vi "writeToXML.vi"(8 "error in (no error)":errorcluster, 10 "ClassLabel":string, 11 "MccAzElMove in":refnum<class "MccAzElMove.lvclass">) -> (0 "error out":errorcluster, 2 "XMLout":string, 3 "MccAzElMove out":refnum<class "MccAzElMove.lvclass">)   [LabVIEW 2022 SP3, in "TCSDataDefinitions.lvlib" / "TCSMountControlCommand.lvlib" / "CommandsForAzElAxes.lvlib" / "MccAzElMove.lvclass"]
uses:
  MccAzElMove.lvclass
  <userlib>/Common/UnitsAndXML/FlattenItemWithUnitToXML/FlattenPlaneAngleToXML/PlaneAngleUnit.ctl
  MccAzElMove.lvclass/MccAzElMove.ctl
  CommandsForAzElAxes.lvclass
  <userlib>/Common/UnitsAndXML/UnitsAndXML.lvlib
  <userlib>/Common/XML/XMLGenerator/XMLGenerator.lvclass
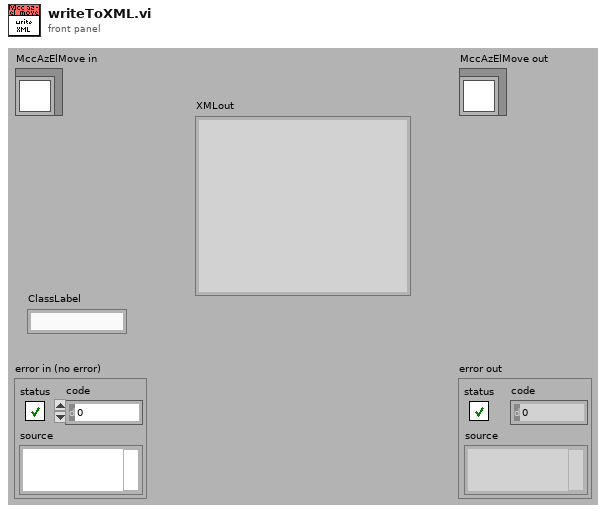
[diagram p1: front panel]
types:
  T1 = typedef "UnitsAndXML.lvlib/PlaneAngleUnit.ctl" = enum16{"rad", "deg", "'", "\""}
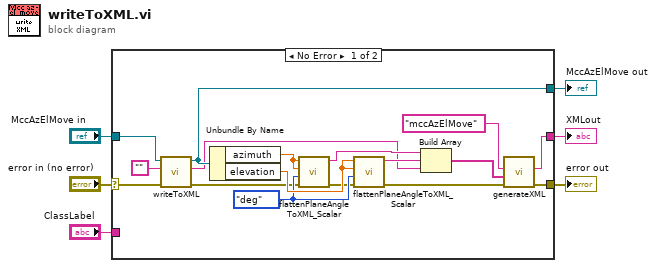
[diagram p0: block diagram]
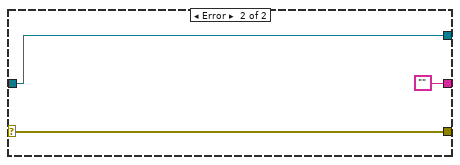
[diagram p2: hidden frame]
diagram:
  n1 = case shown="No Error" "error in (no error)" {
    selector: "error in (no error)" -> [w21 w26]
    tunnel: [w7 w26] -> w5
    tunnel: [w22 w25] -> w3
    tunnel: "MccAzElMove in" -> [w23 w25]
    tunnel: [w9 ""] -> w2
    tunnel: "ClassLabel" -> [_ _]
    frame No Error {
      w18 = PlaneAngleUnit."deg" ("planeAngleUnitInXML")
      n2 = call-parent "writeToXML.vi"("error in (no error)"=w21, "ClassLabel"="", "TCSMCCCommand in"=w23) -> ("error out"=w16:errorcluster, "XMLout"=w13:string, "TCSMCCCommand out"=w22:refnum<class "MccAzElMove.lvclass">)  [unwired: 6 in]
      n3 = Unbundle By Name(w22) -> ("azimuth"=w20:dbl[unit], "elevation"=w19:dbl[unit])
      n4 = call <userlib>:"flattenPlaneAngleToXML_Scalar.vi"("error in (no error)"=w16, "planeAngleUnitInXML"=w18, "planeAngleAgain"=w20, "planeAngle"=w20) -> ("error out"=w17:errorcluster, "xmlString"=w15:string)  [unwired: 6 in]
      n5 = call <userlib>:"flattenPlaneAngleToXML_Scalar.vi"("error in (no error)"=w17, "planeAngleUnitInXML"=w18, "planeAngleAgain"=w19, "planeAngle"=w19) -> ("error out"=w11:errorcluster, "xmlString"=w14:string)  [unwired: 6 in]
      n6 = Build Array(w15, w14, w13) -> (w12:string[])
      n7 = call <userlib>:"generateXML.vi"("error in"=w11, "childrenXML"=w12, "elementName"="mccAzElMove" ("Class Label")) -> ("error out"=w7:errorcluster, "XML out"=w9:string)  [unwired: 6 in, 1 out]
    }
    frame Error {
    }
  }
  "error out" <- w5
  "MccAzElMove out" <- w3
  "XMLout" <- w2
